vi "Proxy_FindDevice.vi"(8 "error in (no error)":errorcluster, 11 "VISA resource":refnum<visa-resource-name>) -> (0 "error out":errorcluster, 3 "VISA resource name out":refnum<visa-resource-name>)   [LabVIEW 2019]
uses:
  <vilib>/Instr/_visa.llb/VISA Configure Serial Port (Instr).vi
  <vilib>/ErrorRing/Error Ring.xnode
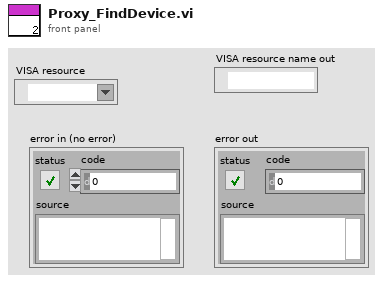
[diagram p1: front panel]
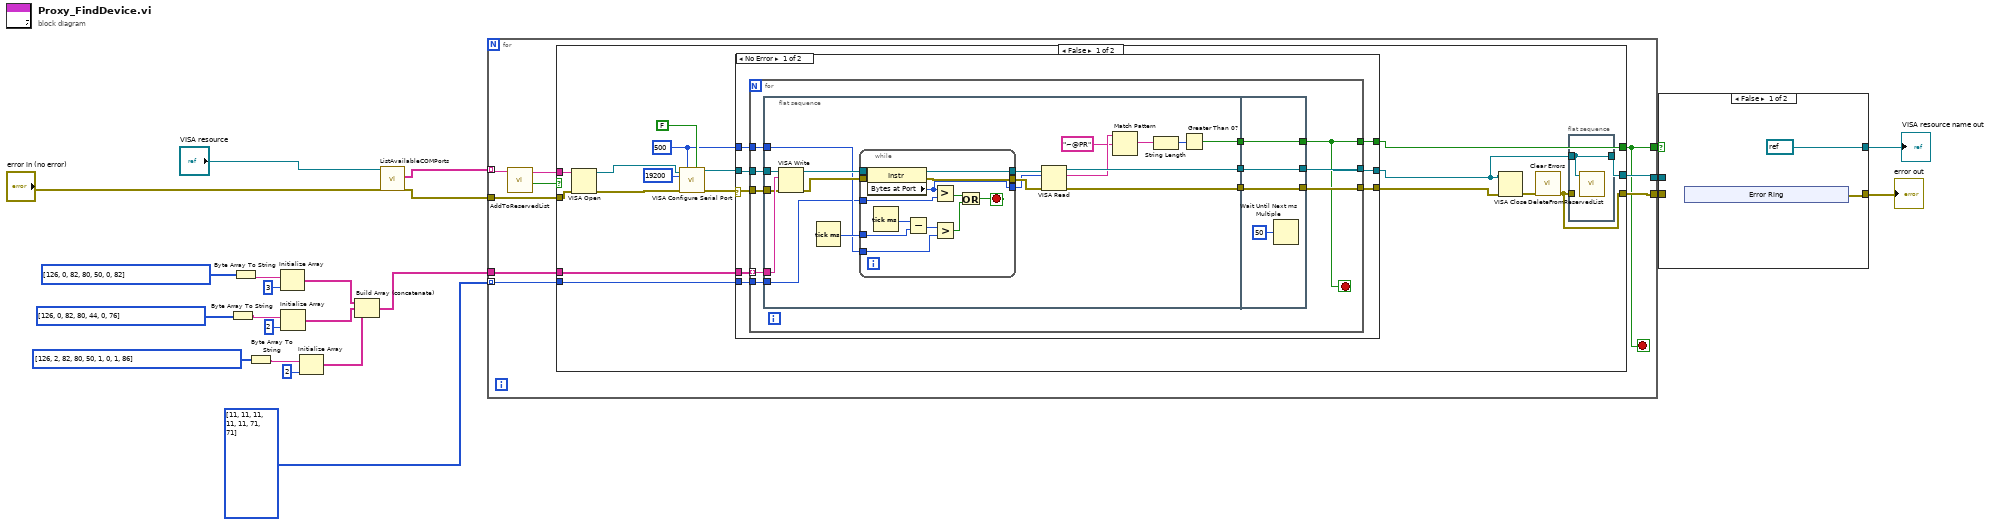
[diagram p0: block diagram]
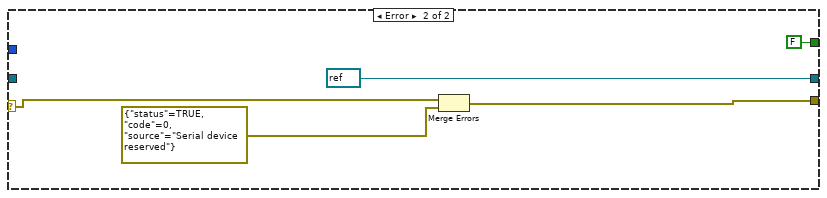
[diagram p3: hidden frame]
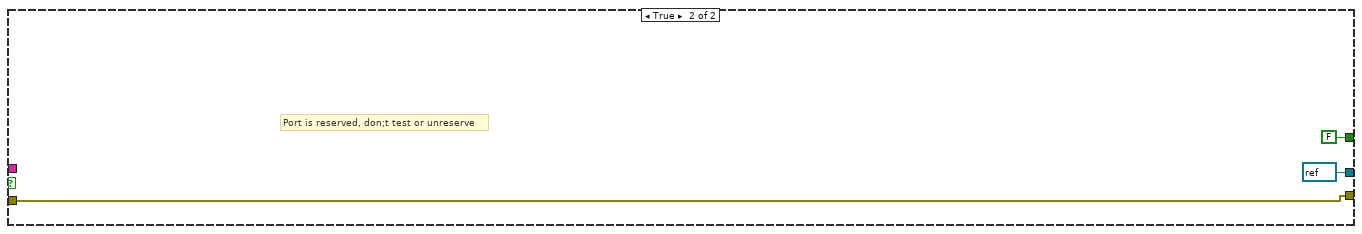
[diagram p4: hidden frame]
diagram:
  n1 = Byte Array To String(unsigned byte array=u8[] [126, 0, 82, 80, 44, 0, 76]) -> (string=w13:string)
  n2 = Byte Array To String(unsigned byte array=u8[] [126, 0, 82, 80, 50, 0, 82]) -> (string=w10:string)
  n3 = Byte Array To String(unsigned byte array=u8[] [126, 2, 82, 80, 50, 1, 0, 1, 86]) -> (string=w14:string)
  n4 = Initialize Array(w10, 3 ("dimension size")) -> (w17:string[])
  n5 = Initialize Array(w13, 2 ("dimension size")) -> (w18:string[])
  n6 = Initialize Array(w14, 2 ("dimension size")) -> (w19:string[])
  n7 = Build Array (concatenate)(w17, w18, w19) -> (w21:string[])
  n8 = call "ListAvailableCOMPorts.vi"("error in (no error)"="error in (no error)", "VISA resource"="VISA resource") -> ("error out"=w20:errorcluster, "Available COM Ports"=w4:string[])  [unwired: 8 in]
  n9 = for {
    tunnel: w4 -> [w32] mode=indexing
    tunnel: w20 -> [w30]
    tunnel: w21 -> [w29]
    tunnel: u16[] [11, 11, 11, 11, 11, 71, 71] -> [w28] mode=indexing
    tunnel: [w27] -> w2
    tunnel: [w26] -> w6
    tunnel: [w24] -> w3
    stop <- w24 stop-if-true
    n10 = call "AddToReservedList.vi"("VISA resource"=w32) -> ("Reserved?"=w25:bool, "VISA resource out"=w31:string)  [unwired: 9 in]
    n11 = case shown="False" w25 {
      tunnel: w31 -> [w49 _]
      tunnel: w30 -> [w47 w110]
      tunnel: w29 -> [w41 _]
      tunnel: w28 -> [w40 _]
      tunnel: [w38 FALSE] -> w24
      tunnel: [w35 w110] -> w27
      tunnel: [w33 refnum<visa-resource-name> refnum ("VISA resource out")] -> w26
      frame False {
        w39 = u32 500 ("timeout (10sec)")
        n12 = VISA Open(error in (no error)=w47, VISA resource name=w49) -> (VISA resource name=w46:refnum<visa-resource-name>, error out=w48:errorcluster)  [unwired: 3 in]
        n13 = call-poly "VISA Configure Serial Port"("VISA resource name"=w46, "timeout (10sec)"=w39, "Enable Termination\nChar (T)"=FALSE ("Enable Termination\nChar (T)"), "baud rate (9600)"=u32 19200, "error in (no error)"=w48) -> ("VISA resource name out"=w42:refnum<visa-resource-name>, "error out"=w43:errorcluster)  [unwired: 9 in]
        n14 = case shown="No Error" w43 {
          selector: w43 -> [w56 w109]
          tunnel: [w53 w107] -> w36
          tunnel: w42 -> [w58 _]
          tunnel: [w52 refnum<visa-resource-name> refnum ("VISA resource name out")] -> w34
          tunnel: w41 -> [w57 _]
          tunnel: w40 -> [w55 _]
          tunnel: w39 -> [w54 _]
          tunnel: [w51 FALSE] -> w38
          frame No Error {
            n15 = for {
              tunnel: w58 -> [w69]
              tunnel: w57 -> [w68] mode=indexing
              tunnel: w56 -> [w67]
              tunnel: w55 -> [w66]
              tunnel: w54 -> [w65]
              tunnel: [w62] -> w53
              tunnel: [w61] -> w52
              tunnel: [w59] -> w51
              stop <- w59 stop-if-true
              n16 = flat-sequence {
                tunnel: w69 -> [w87]
                tunnel: w68 -> [w86]
                tunnel: w67 -> [w85]
                tunnel: w66 -> [w73]
                tunnel: w65 -> [w79]
                tunnel: [w76] -> w64
                tunnel: [w75] -> w63
                tunnel: [w74] -> w60
                tunnel: [w103] -> w59
                tunnel: w64 -> [w103]
                tunnel: w63 -> [w102]
                tunnel: [w102] -> w62
                tunnel: [w101] -> w61
                tunnel: w60 -> [w101]
                frame #0 {
                  n17 = VISA Write(VISA resource name=w87, write buffer=w86, error in (no error)=w85) -> (VISA resource name out=w84:refnum<visa-resource-name>, error out=w83:errorcluster)  [unwired: 1 out]
                  n18 = Tick Count (ms)() -> (millisecond timer value=w80:u32)
                  n19 = while {
                    tunnel: w73 -> [w100]
                    tunnel: w84 -> [w99]
                    tunnel: w83 -> [w98]
                    tunnel: [w97] -> w82
                    tunnel: [w96] -> w81
                    tunnel: w80 -> [w93]
                    tunnel: w79 -> [w91]
                    tunnel: [w88] -> w72
                    stop <- w89 stop-if-true
                    n20 = property class="Instr"(reference=w99, error in=w98) -> (reference out=w97:refnum<visa-resource-name>, error out=w96:errorcluster, "Bytes at Port"=w88:u32)
                    n21 = Tick Count (ms)() -> (millisecond timer value=w94:u32)
                    n22 = Subtract(x=w94, y=w93) -> (x-y=w92:u32)
                    n23 = Greater?(x=w88, y=w100) -> (0:w95:bool)
                    n24 = Greater?(x=w92, y=w91) -> (0:w90:bool)
                    n25 = Or(x=w95, y=w90) -> (x .or. y?=w89:bool)
                  }
                  n26 = VISA Read(VISA resource name=w82, byte count=w72, error in (no error)=w81) -> (VISA resource name out=w74:refnum<visa-resource-name>, read buffer=w71:string, error out=w75:errorcluster)  [unwired: 1 out]
                  n27 = Match Pattern(string=w71, regular expression="~@PR" ("x")) -> (match substring=w78:string)  [unwired: 1 in, 3 out]
                  n28 = String Length(string=w78) -> (length=w77:i32)
                  n29 = Greater Than 0?(x=w77) -> (x > 0?=w76:bool)
                }
                frame #1 {
                  n30 = Wait Until Next ms Multiple(millisecond multiple=u32 50) -> ()  [unwired: 1 out]
                }
              }
            }
          }
          frame Error {
            n31 = Merge Errors(w109, errorcluster {"status"=TRUE, "code"=0, "source"="Serial device reserved"} ("error out")) -> (w107:errorcluster)
          }
        }
        n32 = VISA Close(VISA resource name=w34, error in (no error)=w36) -> (error out=w37:errorcluster)
        n33 = call <vilib>:"Clear Errors.vi"("error in (no error)"=w37) -> ("error out"=w35:errorcluster)  [unwired: 5 in, 1 out]
        n34 = flat-sequence {
          tunnel: w34 -> [w50]
          tunnel: w35 -> [_]
          tunnel: [w50] -> w33
          frame #0 {
            n35 = call "DeleteFromReservedList.vi"("VISA resource"=w50) -> ()  [unwired: 10 in, 1 out]
          }
        }
      }
      frame True {
        # "Port is reserved, don;t test or unreserve"
      }
    }
  }
  n36 = case shown="False" w3 {
    tunnel: w6 -> [_ w117]
    tunnel: [refnum<visa-resource-name> refnum ("VISA resource out") w117] -> w5
    tunnel: w2 -> [_ w116]
    tunnel: [w113 w116] -> w1
    frame False {
      n37 = xnode "Error Ring"() -> ("error out"=w113:errorcluster)
    }
    frame True {
    }
  }
  "VISA resource name out" <- w5
  "error out" <- w1
